vi "Write Limit Current.vi"(8 "error in":errorcluster, 10 "OverCurrent_Protect":dbl, 11 "IF_XX in":refnum<class "IF_XX.lvclass">) -> (0 "error out":errorcluster, 3 "IF_XX out":refnum<class "IF_XX.lvclass">)   [LabVIEW 2019, in "IF_XX.lvlib" / "IF_XX.lvclass"]
uses:
  Library/IF_XX.lvclass
  builds/Instruments/PowerSupply.lvlibp/Library/PowerSupply.lvclass
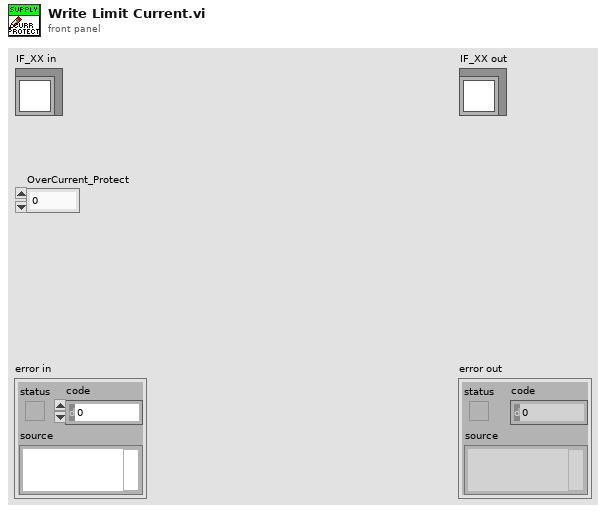
[diagram p1: front panel]
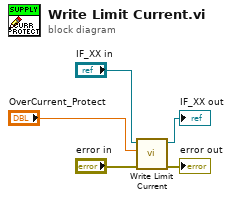
[diagram p0: block diagram]
diagram:
  n1 = call-parent "Write Limit Current.vi"("error in"="error in", "OverCurrent_Protect"="OverCurrent_Protect", "PowerSupply in"="IF_XX in") -> ("error out"=→"error out":errorcluster, "PowerSupply out"=→"IF_XX out":refnum<class "IF_XX.lvclass">)  [unwired: 7 in]
